vi "(C) Save (SubVI).vi"(0 "References":T1, 5 "Step Number":i32, 13 "Strain Values":T2) -> (15 "Save Error":errorcluster)   [LabVIEW 2010]
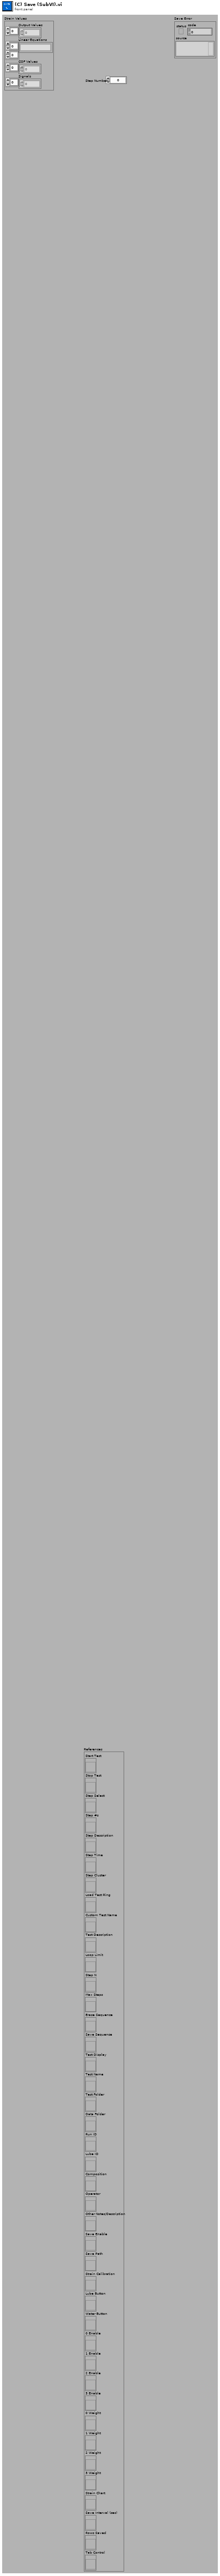
[diagram p1: front panel]
types:
  T1 = cluster{"Start Test":refnum<vi>, "Stop Test":refnum<vi>, "Step Select":refnum<vi>, "Step #s":refnum<vi>, "Step Description":refnum<vi>, "Step Time":refnum<vi>, "Step Cluster":refnum<vi>, "Load Test Ring":refnum<vi>, "Custom Test Name":refnum<vi>, "Test Description":refnum<vi>, "Loop Limit":refnum<vi>, "Step N":refnum<vi>, "Max Steps":refnum<vi>, "Erase Sequence":refnum<vi>, "Save Sequence":refnum<vi>, "Test Display":refnum<vi>, "Test Name":refnum<vi>, "Test Folder":refnum<vi>, "Data Folder":refnum<vi>, "Run ID":refnum<vi>, "Lube ID":refnum<vi>, "Composition":refnum<vi>, "Operator":refnum<vi>, "Other Notes/Description":refnum<vi>, "Save Enable":refnum<vi>, "Save Path":refnum<vi>, "Strain Calibration":refnum<vi>, "Lube Button":refnum<vi>, "Water Button":refnum<vi>, "0 Enable":refnum<vi>, "1 Enable":refnum<vi>, "2 Enable":refnum<vi>, "3 Enable":refnum<vi>, "0 Weight":refnum<vi>, "1 Weight":refnum<vi>, "2 Weight":refnum<vi>, "3 Weight":refnum<vi>, "Strain Chart":refnum<vi>, "Save Interval (sec)":refnum<vi>, "Rows Saved":refnum<vi>, "Tab Control":refnum<vi>}
  T2 = cluster{"Output Values":dbl[], "Linear Equations":string[][], "COF Values":dbl[], "Signals":dbl[]}
  T3 = enum8{"Enabled", "Disabled", "Disabled and Grayed Out"}
  T4 = cluster{"Row Limit":i32, "Default File Name":string, "New File Daily?":bool, "Manual Save Interval?":bool}
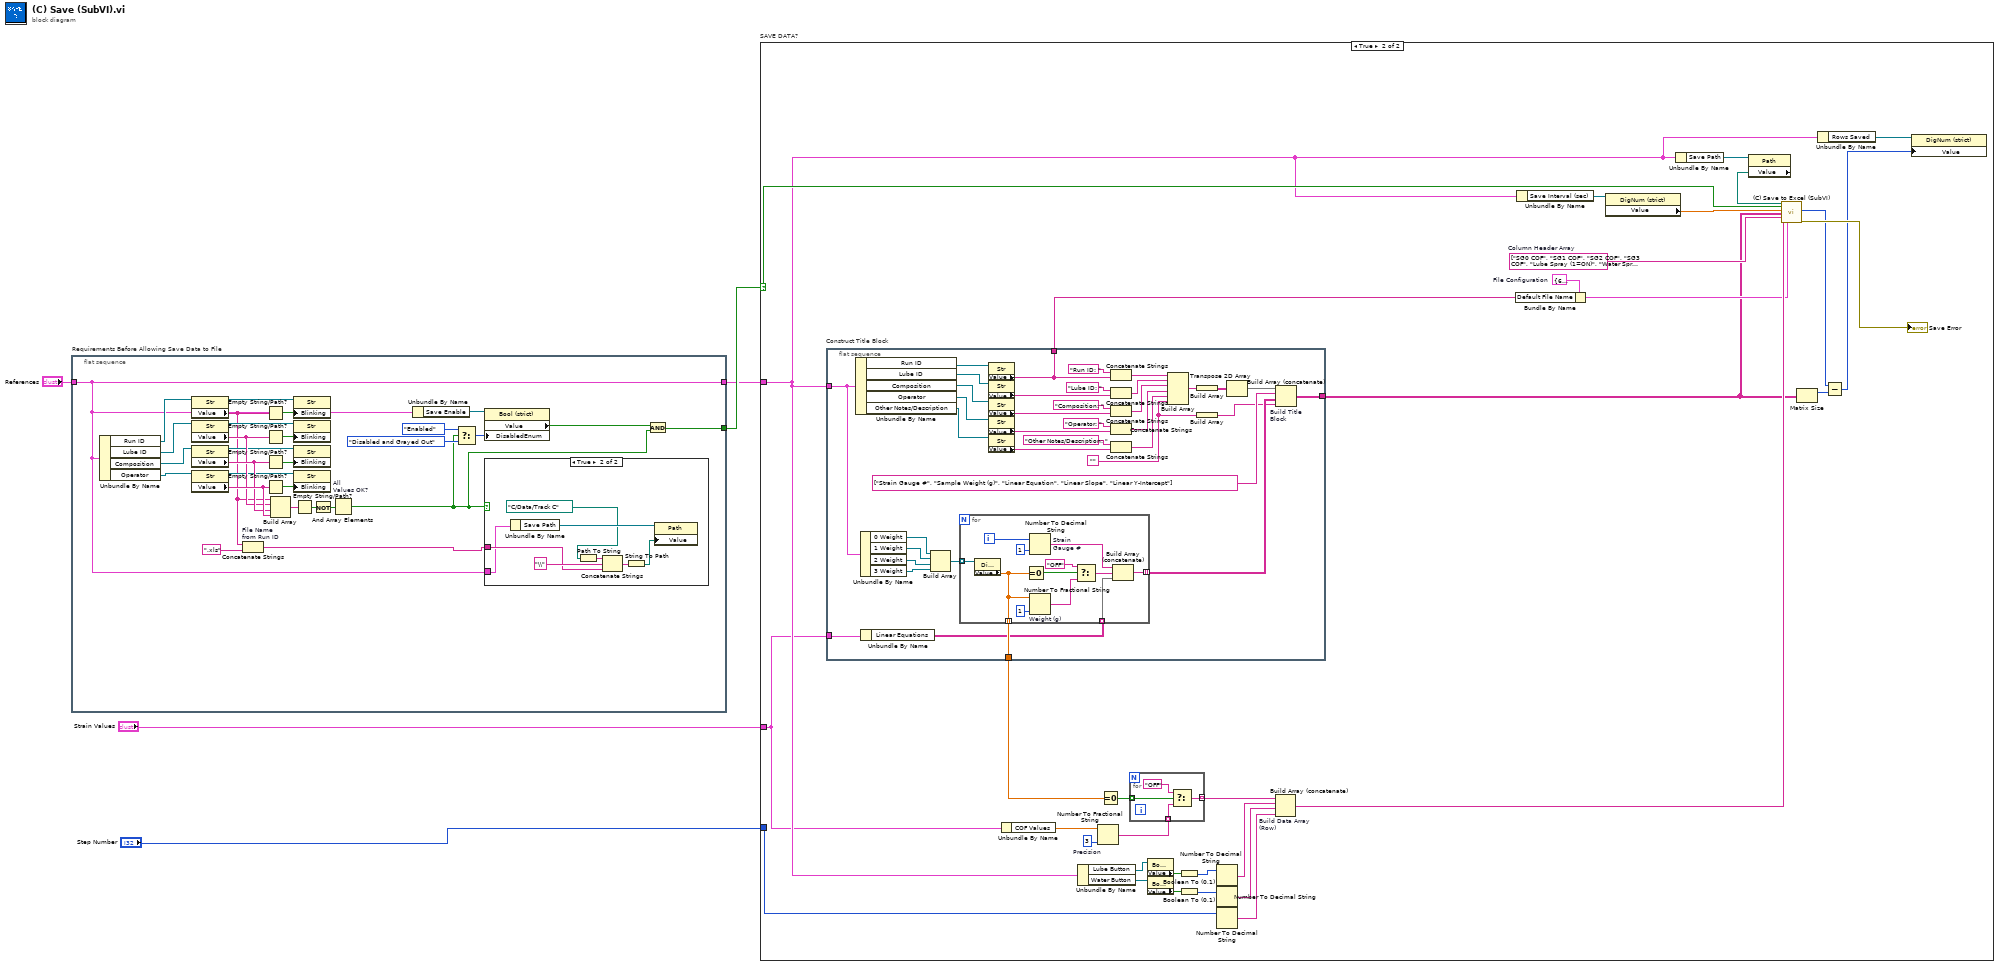
[diagram p0: block diagram]
diagram:
  n1 = flat-sequence "Requirements Before Allowing Save Data to File" {
    tunnel: "References" -> [w7]
    tunnel: [w15] -> w3
    tunnel: [w7] -> w2
    frame #0 {
      n2 = Unbundle By Name(w7) -> ("Run ID"=w18:refnum<vi>, "Lube ID"=w25:refnum<vi>, "Composition"=w28:refnum<vi>, "Operator"=w31:refnum<vi>)
      n3 = property class="Str"(reference=w18) -> (reference out=w16:refnum<vi>, "Value"=w11:string)  [unwired: 1 in, 1 out]
      n4 = property class="Str"(reference=w25) -> (reference out=w24:refnum<vi>, "Value"=w32:string)  [unwired: 1 in, 1 out]
      n5 = property class="Str"(reference=w28) -> (reference out=w27:refnum<vi>, "Value"=w33:string)  [unwired: 1 in, 1 out]
      n6 = property class="Str"(reference=w31) -> (reference out=w30:refnum<vi>, "Value"=w34:string)  [unwired: 1 in, 1 out]
      n7 = Concatenate Strings "File Name\nfrom Run ID"(w11, ".xls") -> (w8:string)
      n8 = Empty String/Path?(string/path=w11) -> (empty?=w22:bool)
      n9 = Empty String/Path?(string/path=w32) -> (empty?=w23:bool)
      n10 = Empty String/Path?(string/path=w33) -> (empty?=w26:bool)
      n11 = Empty String/Path?(string/path=w34) -> (empty?=w29:bool)
      n12 = Build Array(w11, w32, w33, w34) -> (w21:string[])
      n13 = property class="Str"(reference=w16, "Blinking"=w22) -> ()  [unwired: 1 in, 2 out]
      n14 = property class="Str"(reference=w24, "Blinking"=w23) -> ()  [unwired: 1 in, 2 out]
      n15 = property class="Str"(reference=w27, "Blinking"=w26) -> ()  [unwired: 1 in, 2 out]
      n16 = property class="Str"(reference=w30, "Blinking"=w29) -> ()  [unwired: 1 in, 2 out]
      n17 = Empty String/Path?(string/path=w21) -> (empty?=w19:bool[])
      n18 = Not(x=w19) -> (.not. x?=w20:bool[])
      n19 = And Array Elements "All\nValues OK?"(Boolean array=w20) -> (logical AND=w6:bool)
      n20 = Unbundle By Name(w7) -> ("Save Enable"=w17:refnum<vi>)
      n21 = Select(t=T3."Enabled" ("Disabled"), s=w6, f=T3."Disabled and Grayed Out" ("Disabled")) -> (s? t:f=w10:T3)
      n22 = property class="Bool (strict)"(reference=w17, "DisabledEnum"=w10) -> ("Value"=w9:bool)  [unwired: 1 in, 2 out]
      n23 = case shown="True" w6 {
        tunnel: w8 -> [_ w38]
        tunnel: w7 -> [_ w36]
        frame False {
        }
        frame True {
          n24 = Unbundle By Name(w36) -> ("Save Path"=w42:refnum<vi>)
          n25 = Path To String(path=path "C:/Data/Track C") -> (string=w41:string)
          n26 = Concatenate Strings(w41, "\\" ("string"), w38) -> (w40:string)
          n27 = String To Path(string=w40) -> (path=w37:path)
          n28 = property class="Path"(reference=w42, "Value"=w37) -> ()  [unwired: 1 in, 2 out]
        }
      }
      n29 = And(x=w9, y=w6) -> (x .and. y?=w15:bool)
    }
  }
  n30 = case "SAVE DATA?" shown="True" w3 {
    selector: w3 -> [_ w46]
    tunnel: "Step Number" -> [_ w68]
    tunnel: "Strain Values" -> [_ w43]
    tunnel: w2 -> [_ w45]
    frame False {
    }
    frame True {
      w67 = i16 3  # Precision
      w75 = string[] ["SG0 COF", "SG1 COF", "SG2 COF", "SG3 COF", "Lube Spray (1=ON)", "Water Spray (1=ON)", "Test Step"]  # Column Header Array
      w76 = T4 {"Row Limit"=65500, "Default File Name"="Default", "New File Daily?"=FALSE, "Manual Save Interval?"=FALSE}  # File Configuration
      n31 = flat-sequence "Construct Title Block" {
        tunnel: [w82] -> w57
        tunnel: [w81] -> w54
        tunnel: [w80] -> w52
        tunnel: w45 -> [w79]
        tunnel: w43 -> [w78]
        frame #0 {
          w91 = ""
          n32 = Unbundle By Name(w79) -> ("Run ID"=w90:refnum<vi>, "Lube ID"=w89:refnum<vi>, "Composition"=w88:refnum<vi>, "Operator"=w87:refnum<vi>, "Other Notes/Description"=w86:refnum<vi>)
          n33 = Unbundle By Name(w79) -> ("0 Weight"=w113:refnum<vi>, "1 Weight"=w112:refnum<vi>, "2 Weight"=w111:refnum<vi>, "3 Weight"=w110:refnum<vi>)
          n34 = Unbundle By Name(w78) -> ("Linear Equations"=w77:string[][])
          n35 = Build Array(w113, w112, w111, w110) -> (w109:refnum<vi>[])
          n36 = for {
            tunnel: w109 -> [w121] mode=indexing
            tunnel: [w122] -> w107 mode=indexing
            tunnel: [w118] -> w81 mode=indexing
            tunnel: w77 -> [w120] mode=indexing
            i -> [w114]
            n37 = property class="DigNum (strict)"(reference=w121) -> ("Value"=w118:dbl)  [unwired: 1 in, 2 out]
            n38 = Equal To 0?(x=w118) -> (x = 0?=w117:bool)
            n39 = Number To Decimal String "Strain\nGauge #"(number=w114, width (-)=i16 1) -> (decimal integer string=w123:string)
            n40 = Number To Fractional String "Weight (g)"(number=w118, precision (6)=i16 1) -> (F-format string=w116:string)  [unwired: 2 in]
            n41 = Select(t="OFF" ("string"), s=w117, f=w116) -> (s? t:f=w115:string)
            n42 = Build Array (concatenate)(w123, w115, w120) -> (w122:string[])
          }
          n43 = property class="Str"(reference=w90) -> ("Value"=w82:string)  [unwired: 1 in, 2 out]
          n44 = property class="Str"(reference=w89) -> ("Value"=w85:string)  [unwired: 1 in, 2 out]
          n45 = property class="Str"(reference=w88) -> ("Value"=w84:string)  [unwired: 1 in, 2 out]
          n46 = property class="Str"(reference=w87) -> ("Value"=w83:string)  [unwired: 1 in, 2 out]
          n47 = property class="Str"(reference=w86) -> ("Value"=w100:string)  [unwired: 1 in, 2 out]
          n48 = Concatenate Strings("Run ID: " ("string"), w82) -> (w99:string)
          n49 = Concatenate Strings("Lube ID: " ("string"), w85) -> (w98:string)
          n50 = Concatenate Strings("Composition: " ("string"), w84) -> (w97:string)
          n51 = Concatenate Strings("Operator: " ("string"), w83) -> (w96:string)
          n52 = Concatenate Strings("Other Notes/Description: " ("string"), w100) -> (w95:string)
          n53 = Build Array(w99, w98, w97, w96, w95, w91) -> (w94:string[])
          n54 = Build Array(w94) -> (w93:string[][])
          n55 = Build Array(w91) -> (w106:string[])
          n56 = Transpose 2D Array(2D array=w93) -> (transposed array=w92:string[][])
          n57 = Build Array (concatenate) "Build Title\nBlock"(w92, string[] ["Strain Gauge #", "Sample Weight (g)", "Linear Equation", "Linear Slope", "Linear Y-Intercept"], w107, w106) -> (w80:string[][])
        }
      }
      n58 = Unbundle By Name(w43) -> ("COF Values"=w58:dbl[])
      n59 = Unbundle By Name(w45) -> ("Lube Button"=w74:refnum<vi>, "Water Button"=w73:refnum<vi>)
      n60 = Number To Fractional String(number=w58, precision (6)=w67) -> (F-format string=w62:string[])  [unwired: 2 in]
      n61 = Equal To 0?(x=w54) -> (x = 0?=w53:bool[])
      n62 = for {
        tunnel: w62 -> [w128] mode=indexing
        tunnel: [w127] -> w61 mode=indexing
        tunnel: w53 -> [w126] mode=indexing
        n63 = Select(t="OFF" ("string"), s=w126, f=w128) -> (s? t:f=w127:string)
      }
      n64 = property class="Bool (strict)"(reference=w74) -> ("Value"=w72:bool)  [unwired: 1 in, 2 out]
      n65 = property class="Bool (strict)"(reference=w73) -> ("Value"=w71:bool)  [unwired: 1 in, 2 out]
      n66 = Boolean To (0,1)(Boolean=w72) -> (0, 1=w70:i16)
      n67 = Boolean To (0,1)(Boolean=w71) -> (0, 1=w69:i16)
      n68 = Number To Decimal String(number=w70) -> (decimal integer string=w66:string)  [unwired: 1 in]
      n69 = Number To Decimal String(number=w69) -> (decimal integer string=w65:string)  [unwired: 1 in]
      n70 = Number To Decimal String(number=w68) -> (decimal integer string=w64:string)  [unwired: 1 in]
      n71 = Build Array (concatenate) "Build Data Array\n(Row)"(w61, w66, w65, w64) -> (w63:string[])
      n72 = Bundle By Name(cluster=w76, "Default File Name"=w57) -> (w60:T4)
      n73 = Unbundle By Name(w45) -> ("Save Interval (sec)"=w49:refnum<vi>)
      n74 = property class="DigNum (strict)"(reference=w49) -> ("Value"=w48:dbl)  [unwired: 1 in, 2 out]
      n75 = Unbundle By Name(w45) -> ("Save Path"=w55:refnum<vi>)
      n76 = property class="Path"(reference=w55) -> ("Value"=w56:path)  [unwired: 1 in, 2 out]
      n77 = call "(C) Save to Excel (SubVI).vi"("File Path Input"=w56, "Save (Enable/Signal)"=w46, "Save Interval (s)"=w48, "Title Block"=w52, "Column Header Array"=w75, "Data Array (Row)"=w63, "File Configuration"=w60) -> ("# of Rows Saved"=w50:i32, "Error Output"=→"Save Error":errorcluster)  [unwired: 8 in, 3 out]
      n78 = Matrix Size(0:w52) -> (1:w51:i32)  [unwired: 1 out]
      n79 = Unbundle By Name(w45) -> ("Rows Saved"=w47:refnum<vi>)
      n80 = Subtract(x=w50, y=w51) -> (x-y=w44:i32)
      n81 = property class="DigNum (strict)"(reference=w47, "Value"=w44) -> ()  [unwired: 1 in, 2 out]
    }
  }
